vi "Store Actors.vi"(8 "error in (no error)":errorcluster, 9 "Actor Paths":path[](array[path]), 10 "Actors":string[](array[string]), 11 "Target Store in":refnum<class "Target Store.lvclass">) -> (0 "error out":errorcluster, 3 "Target Store out":refnum<class "Target Store.lvclass">)   [LabVIEW 2023, in "Add Actor.lvlib" / "Target Store.lvclass"]
uses:
  Target Store.lvclass
  Target Store.lvclass/Target Store.ctl
  AFPP Shared/Constants.vi
  AFPP Shared/AFPP Shared.lvlib
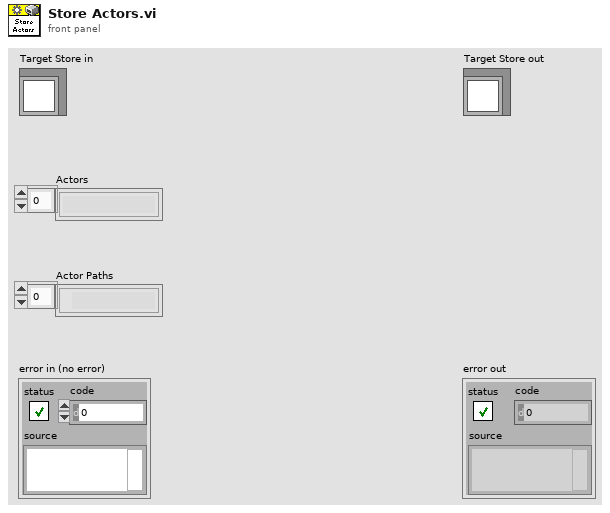
[diagram p1: front panel]
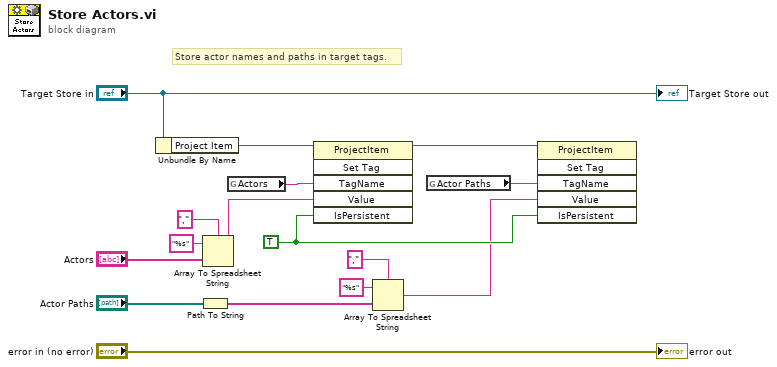
[diagram p0: block diagram]
diagram:
  w10 = TRUE ("Is Persistent")
  # "Store actor names and paths in target tags."
  n1 = Unbundle By Name("Target Store in") -> ("Project Item"=w12:refnum<vi>)
  n2 = Path To String(path="Actor Paths") -> (string=w4:string[])
  n3 = Array To Spreadsheet String(delimiter (Tab)=",", array="Actors", 3:"%s" ("format string")) -> (spreadsheet string=w7:string)
  n4 = global read "Constants.vi" "Actors"() -> (w2:string)
  n5 = invoke class="ProjectItem" method="Set Tag"(reference=w12, "TagName"=w2, "Value"=w7, "IsPersistent"=w10) -> (reference out=w11:refnum<vi>)  [unwired: 2 in, 5 out]
  n6 = Array To Spreadsheet String(delimiter (Tab)=",", array=w4, 3:"%s" ("format string")) -> (spreadsheet string=w3:string)
  n7 = global read "Constants.vi" "Actor Paths"() -> (w1:string)
  n8 = invoke class="ProjectItem" method="Set Tag"(reference=w11, "TagName"=w1, "Value"=w3, "IsPersistent"=w10) -> ()  [unwired: 2 in, 6 out]
  "error out" <- "error in (no error)"
  "Target Store out" <- "Target Store in"
